vi "handle FP.vi"(8 "error in (no error)":errorcluster, 11 "VI Refnum":refnum<vi>) -> (0 "error out":errorcluster)   [LabVIEW 2018]
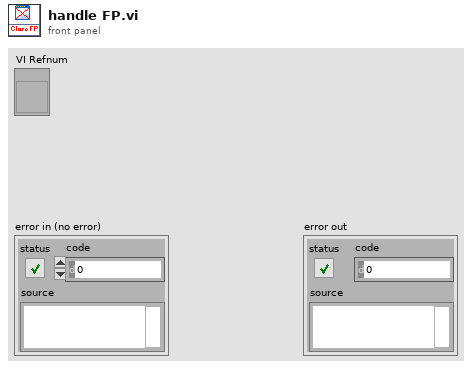
[diagram p1: front panel]
types:
  T1 = enum32{"invalid app kind", "Development System", "Run Time System", "Student Edition", "Embedded LabVIEW", "Evaluation", "Custom"}
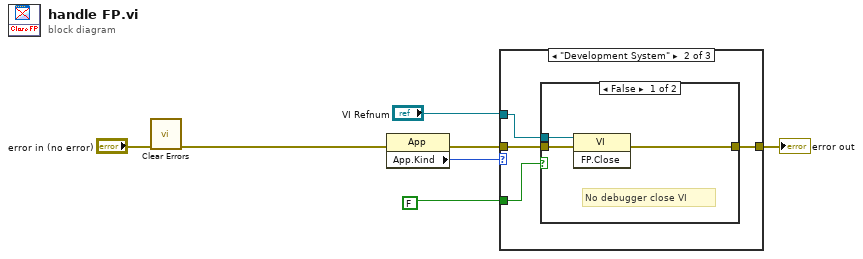
[diagram p0: block diagram]
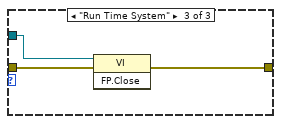
[diagram p4: hidden frame]
diagram:
  n1 = call <vilib>:"Clear Errors.vi"("error in (no error)"="error in (no error)") -> ("error out"=w2:errorcluster)  [unwired: 5 in, 1 out]
  n2 = property class="App"(error in=w2) -> (error out=w5:errorcluster, "App.Kind"=w7:T1)  [unwired: 1 in, 1 out]
  n3 = case shown="\"Development System\"" w7 {
    tunnel: "VI Refnum" -> [_ w10 w19]
    tunnel: w5 -> [w8 w12 w18]
    tunnel: [w8 w11 w17] -> w4
    tunnel: FALSE -> [_ w9 _]
    frame "invalid app kind", Default {
    }
    frame "Development System" {
      n4 = case shown="False" w9 {
        tunnel: w12 -> [w15 w16]
        tunnel: [w14 w16] -> w11
        tunnel: w10 -> [w13 _]
        frame False {
          # "No debugger close VI"
          n5 = invoke class="VI" method="FP.Close"(reference=w13, error in=w15) -> (error out=w14:errorcluster)  [unwired: 1 in, 2 out]
        }
        frame True {
          # "Dont Close VI \nas Debugging is on"
        }
      }
    }
    frame "Run Time System" {
      n6 = invoke class="VI" method="FP.Close"(reference=w19, error in=w18) -> (error out=w17:errorcluster)  [unwired: 1 in, 2 out]
    }
  }
  "error out" <- w4
